vi "Start RunService.vi"(8 "error in (no error)":errorcluster, 11 "project folder":path) -> (0 "error out":errorcluster, 3 "project folder out":path)   [LabVIEW 2019]
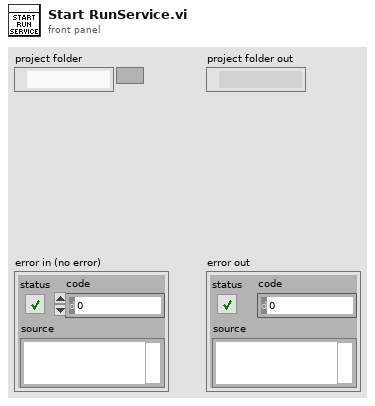
[diagram p1: front panel]
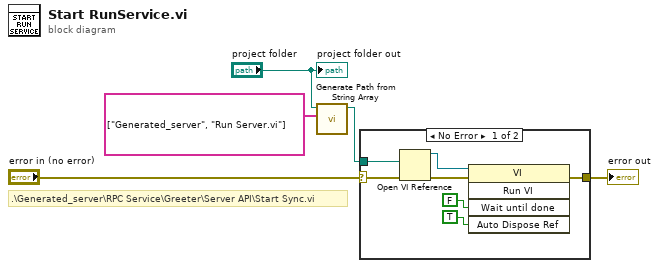
[diagram p0: block diagram]
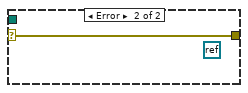
[diagram p2: hidden frame]
diagram:
  # ".\\Generated_server\\RPC Service\\Greeter\\Server API\\Start Sync.vi"
  n1 = call "Generate Path from String Array.vi"("String Array"=string[] ["Generated_server", "Run Server.vi"], "Base Path"="project folder") -> ("project folder out"=w2:path)  [unwired: 9 in]
  n2 = case shown="No Error" "error in (no error)" {
    selector: "error in (no error)" -> [w11 w13]
    tunnel: w2 -> [w12 _]
    tunnel: [w8 w13] -> w1
    frame No Error {
      n3 = Open VI Reference(vi path=w12, error in (no error)=w11) -> (vi reference=w10:refnum<vi>, error out=w9:errorcluster)  [unwired: 4 in]
      n4 = invoke class="VI" method="Run VI"(reference=w10, error in=w9, "Wait until done"=FALSE ("Auto Dispose Reference"), "Auto Dispose Ref"=TRUE ("Auto Dispose Reference")) -> (error out=w8:errorcluster)  [unwired: 1 in, 4 out]
    }
    frame Error {
      (unwired) refnum<k0> refnum
    }
  }
  "error out" <- w1
  "project folder out" <- "project folder"
